vi "SOUR_POW_CORR_COLL_TABL_SEL.vi"(0 "VISA IN":refnum<visa-resource-name>, 1 "Cal Factor Table":string, 5 "error in":errorcluster, 7 "Channel":i32) -> (14 "VISA Out":refnum<visa-resource-name>, 19 "error out":errorcluster)   [LabVIEW 2018, in "PNA-X.lvlib"]
doc: "SOURce<cnum>:POWer:CORRection:COLLect:TABLe[:SELect] <char> \n1845\n\n(Read-Write) Selects which table you want to write to or read from. Read or write using \nSOURce:POWer:CORRection:COLLect:TABLe:FREQuency and \nSOURce:POWer:CORRection:COLLect:TABLe:DATA \nParameters \n<cnum> Any existing channel number. If unspecified, value is set to 1 \n<char> Choose from: \nNONE - No table selected \nASENsor - Cal Factor table for Power Sensor A \nBSENsor - Cal Factor table for Power Sensor B \nLOSS - Loss compensation table \nExamples SOUR:POW:CORR:COLL:TABL ASEN \nsource1:power2:correction:collect:table:select bsensor \nQuery Syntax SOURce:POWer:CORRection:COLLect:TABLe[:SELect]? \nReturn Type Character \nDefault NONE"
uses:
  PNA-X.lvlib
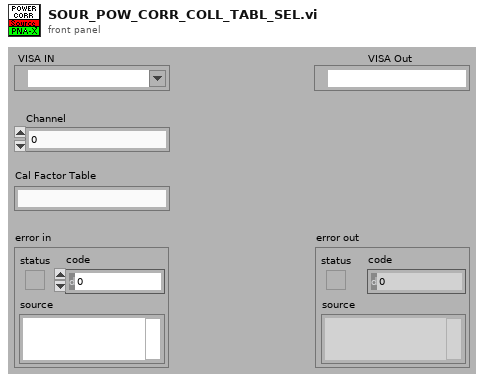
[diagram p1: front panel]
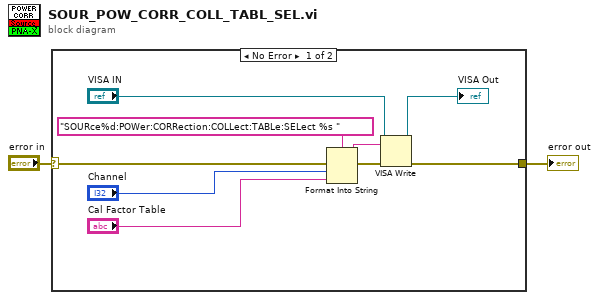
[diagram p0: block diagram]
diagram:
  n1 = case shown="No Error" "error in" {
    selector: "error in" -> [w11 w12]
    tunnel: [w6 w12] -> w1
    frame No Error {
      n2 = Format Into String(format string="SOURce%d:POWer:CORRection:COLLect:TABLe:SELect %s " ("Cmdline"), error in=w11, "Channel", "Cal Factor Table") -> (resulting string=w9:string, error out=w10:errorcluster)  [unwired: 1 in]
      n3 = VISA Write(VISA resource name="VISA IN", write buffer=w9, error in (no error)=w10) -> (VISA resource name out=→"VISA Out":refnum<visa-resource-name>, error out=w6:errorcluster)  [unwired: 1 out]
    }
    frame Error {
    }
  }
  "error out" <- w1
